vi "Plot Editor_Plot to Data & Controls.vi"(6 "Control Refnums":refnum<vi>[](array[refnum]), 7 "XYGraph in":refnum<vi>, 8 "error in (no error)":errorcluster, 11 "Plot Editor Internal Data in":T1) -> (0 "error out":errorcluster, 3 "Plot Editor Internal Data out":T1)   [LabVIEW 2019, in "Plot Editor.lvlib"]
uses:
  Plot Editor.lvlib
  Plot Editor Internal Variables.ctl
  XY Graph/XY Graph Plot Properties.ctl
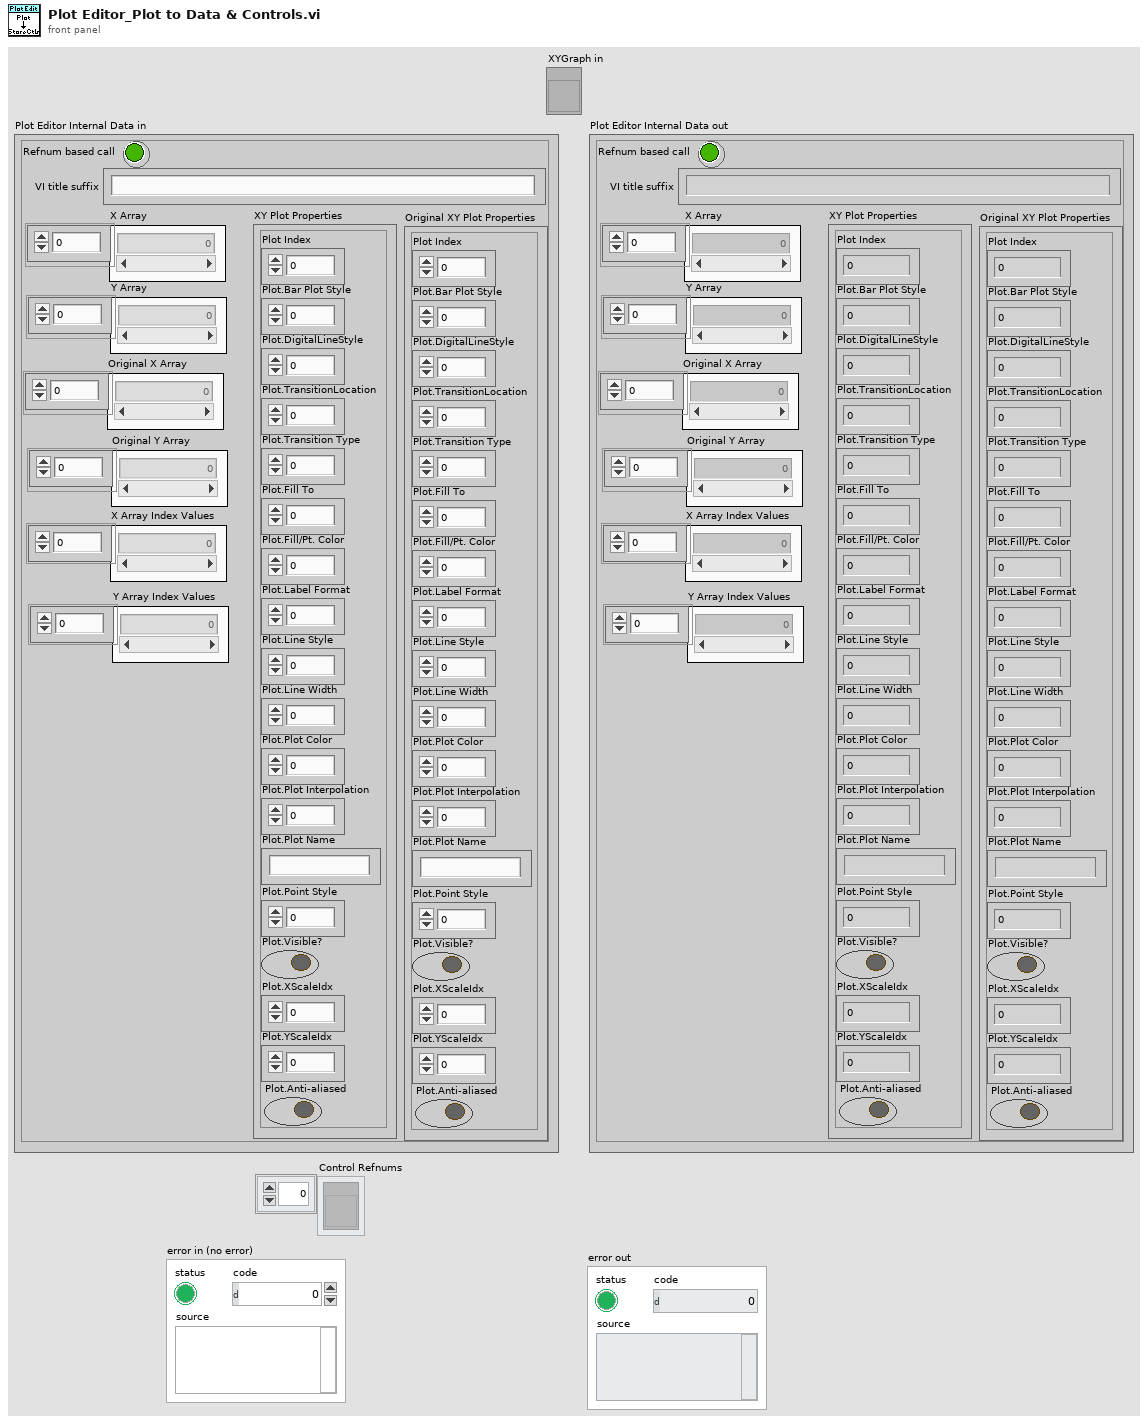
[diagram p1: front panel]
types:
  T1 = typedef "Plot Editor.lvlib/Plot Editor Internal Variables.ctl" = cluster{"X Array":dbl[], "Y Array":dbl[], "XY Plot Properties":T2, "X Array Index Values":u32[], "Y Array Index Values":u32[], "Original XY Plot Properties":T2, "Original X Array":dbl[], "Original Y Array":dbl[], "VI title suffix":string, "Refnum based call":bool}
  T2 = typedef "XY Graph Plot Properties.ctl" = cluster{"Plot Index":i32, "Plot.Bar Plot Style":u8, "Plot.DigitalLineStyle":u8, "Plot.TransitionLocation":u8, "Plot.Transition Type":u8, "Plot.Fill To":i16, "Plot.Fill/Pt. Color":u32, "Plot.Label Format":u8, "Plot.Line Style":u8, "Plot.Line Width":u8, "Plot.Plot Color":u32, "Plot.Plot Interpolation":u8, "Plot.Plot Name":string, "Plot.Point Style":u8, "Plot.Visible?":bool, "Plot.XScaleIdx":u32, "Plot.YScaleIdx":u32, "Plot.Anti-aliased":bool}
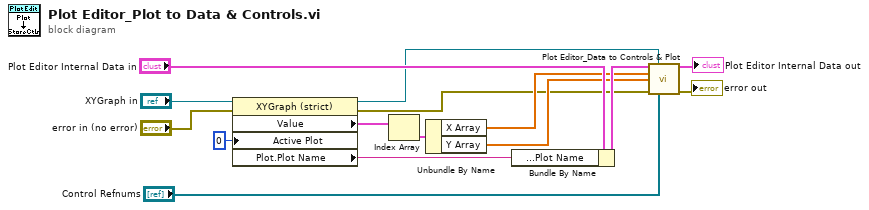
[diagram p0: block diagram]
diagram:
  n1 = property class="XYGraph (strict)"(reference="XYGraph in", error in="error in (no error)", "Active Plot"=u32 0) -> (reference out=w5:refnum<vi>, error out=w3:errorcluster, "Value"=w12:cluster{"X Array":dbl[], "Y Array":dbl[]}[], "Plot.Plot Name"=w9:string)
  n2 = Index Array(array=w12) -> (element=w11:cluster{"X Array":dbl[], "Y Array":dbl[]})  [unwired: 1 in]
  n3 = Unbundle By Name(w11) -> ("X Array"=w7:dbl[], "Y Array"=w6:dbl[])
  n4 = Bundle By Name(cluster="Plot Editor Internal Data in", "XY Plot Properties.Plot.Plot Name"=w9) -> (w8:T1)
  n5 = call "Plot Editor_Data to Controls & Plot.vi"("Plot Editor Internal Data"=w8, "XYGraph in"=w5, "X Array"=w7, "Y Array"=w6, "error in (no error)"=w3, "Control Refnums"="Control Refnums") -> ("Plot Editor Internal Data"=→"Plot Editor Internal Data out":T1, "error out"=→"error out":errorcluster)  [unwired: 8 in]
